vi "Begin.vi"() -> (0 "error in":errorcluster)   [LabVIEW 2013]
doc: "Called before other user functions, this VI is expected to open initial I/O refnums, load in file data, and do all program initialization. Notice that the <B>error out</B> terminal is simply used for data flow. Wiring it to other structures or subVIs ensures that this VI runs first."
uses:
  <vilib>/Rock Robotics/WPI/Joystick/WPI_JoystickDeviceEnum.ctl
  <vilib>/Rock Robotics/SystemInterfaces/DIO/FPGA_DIOPWMChannel.ctl
  <vilib>/Rock Robotics/SystemInterfaces/AI/FPGA_AIChannel.ctl
  <vilib>/Rock Robotics/SystemInterfaces/Typedef/FPGA_TypedefAnalogModule.ctl
  <vilib>/Rock Robotics/SystemInterfaces/DIO/FPGA_DIOChannel.ctl
  <vilib>/Rock Robotics/WPI/Encoder/WPI_EncoderType.ctl
  <vilib>/Rock Robotics/WPI/RobotDrive/WPI_RobotDriveOpen2MotorWithTalon.vi
  <vilib>/Rock Robotics/WPI/MotorControl/WPI_MotorControlOpen Talon.vi
  <vilib>/Rock Robotics/WPI/Counter/WPI_CounterDigitalInputToDigitalSource.vi
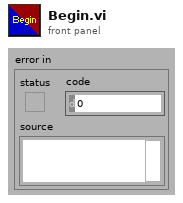
[diagram p1: front panel]
types:
  T1 = typedef "FPGA_DIOPWMChannel.ctl" = enum8{"PWM 1", "PWM 2", "PWM 3", "PWM 4", "PWM 5", "PWM 6", "PWM 7", "PWM 8", "PWM 9", "PWM 10", "Invalid"}
  T2 = typedef "WPI_JoystickDeviceEnum.ctl" = enum16{"USB 1", "USB 2", "USB 3", "USB 4", "Kinect 1", "Kinect 2"}
  T3 = typedef "FPGA_DIOChannel.ctl" = enum8{"DIO 1", "DIO 2", "DIO 3", "DIO 4", "DIO 5", "DIO 6", "DIO 7", "DIO 8", "DIO 9", "DIO 10", "DIO 11", "DIO 12", "DIO 13", "DIO 14", "Invalid"}
  T4 = typedef "WPI_EncoderType.ctl" = enum16{"1x", "2x", "4x"}
  T5 = typedef "FPGA_AIChannel.ctl" = enum8{"AI 1", "AI 2", "AI 3", "AI 4", "AI 5", "AI 6", "AI 7", "AI 8", "Invalid"}
  T6 = typedef "FPGA_TypedefAnalogModule.ctl" = enum16{"Analog Module 1", "Analog Module 2"}
  T7 = typedef "WPI_RobotDriveDevRef.ctl" = cluster{"DevStatus":errorcluster, "Motors[]":T8[], "Square Inputs":bool, "Max Output":dbl, "Isochronous":bool}
  T8 = typedef "WPI_MotorControlDeviceRef.ctl" = cluster{"DeviceStatus":errorcluster, "Type":enum16{"PWM", "CAN"}, "PWM":cluster{"Digital Module":T9, "PWM Channel":T1, "DeadBand":T10}, "CAN":cluster{"Device Number":u8, "Control Mode":T11, "Semaphore":T12, "Max Vout":dbl}, "Invert":bool, "TransformRef":T13, "InvTransformRef":T13}
  T9 = typedef "FPGA_TypedefDigitalModule.ctl" = enum16{"Digital Module 1", "Digital Module 2"}
  T10 = typedef "WPI_PWMDeadband.ctl" = cluster{"Name":string, "maxPositivePwm":i32, "minPositivePwm":i32, "centerPwm":i32, "maxNegativePwm":i32, "minNegativePwm":i32, "angularRange":u16}
  T11 = typedef "WPI_CANJaguar_ControlMode.ctl" = enum8{"Percent VBus", "Current", "Speed", "Position", "Voltage"}
  T12 = typedef "Semaphore RefNum" = refnum<k1>
  T13 = typedef "WPI_PWMTransform_ConPane.ctl" = refnum<vi>
  T14 = typedef "WPI_AnalogChannelDevRef.ctl" = cluster{"DevStatus":errorcluster, "Analog Module":T6, "Analog Channel":T5}
  T15 = typedef "WPI_DigitalInputDevRef.ctl" = cluster{"DevStatus":errorcluster, "DIO Channel":T3, "Digital Module":T9}
  T16 = typedef "FPGA_CounterEncoderSourceConvertionLVSourceType.ctl" = cluster{"DevStatus":errorcluster, "AnalogTriggerMode?":bool, "DigitalMode":cluster{"Digital Module":T9, "DIO Channel":T17}, "AnalogTriggerMode":cluster{"AnalogTriggerIndex":T18, "OutputType":T19}}
  T17 = typedef "FPGA_DIODigitalSourceChannel.ctl" = enum8{"DIO 1", "DIO 2", "DIO 3", "DIO 4", "DIO 5", "DIO 6", "DIO 7", "DIO 8", "DIO 9", "DIO 10", "DIO 11", "DIO 12", "DIO 13", "DIO 14", "Disabled"}
  T18 = typedef "FPGA_AnalogTriggerIndex.ctl" = enum8{"Trig 0", "Trig 1", "Trig 2", "Trig 3", "Trig 4", "Trig 5", "Trig 6", "Trig 7", "Invalid"}
  T19 = typedef "FPGA_AnalogTriggerOutType.ctl" = enum16{"InWindow", "TriggerState", "Rising", "Falling"}
  T20 = typedef "WPI_EncoderDevRef.ctl" = cluster{"DevStatus":errorcluster, "EncoderIndex":T21, "CounterIndex":T22, "DistancePerCount":dbl, "Decoding Type":T4}
  T21 = typedef "FPGA_EncoderIdx.ctl" = enum8{"Enc 0", "Enc 1", "Enc 2", "Enc 3", "Invalid"}
  T22 = typedef "FPGA_CounterCtrSystemIndex.ctl" = enum8{"Ctr 0", "Ctr 1", "Ctr 2", "Ctr 3", "Ctr 4", "Ctr 5", "Ctr 6", "Ctr 7", "Invalid"}
  T23 = typedef "WPI_JoystickDevRef.ctl" = cluster{"Device":T2}
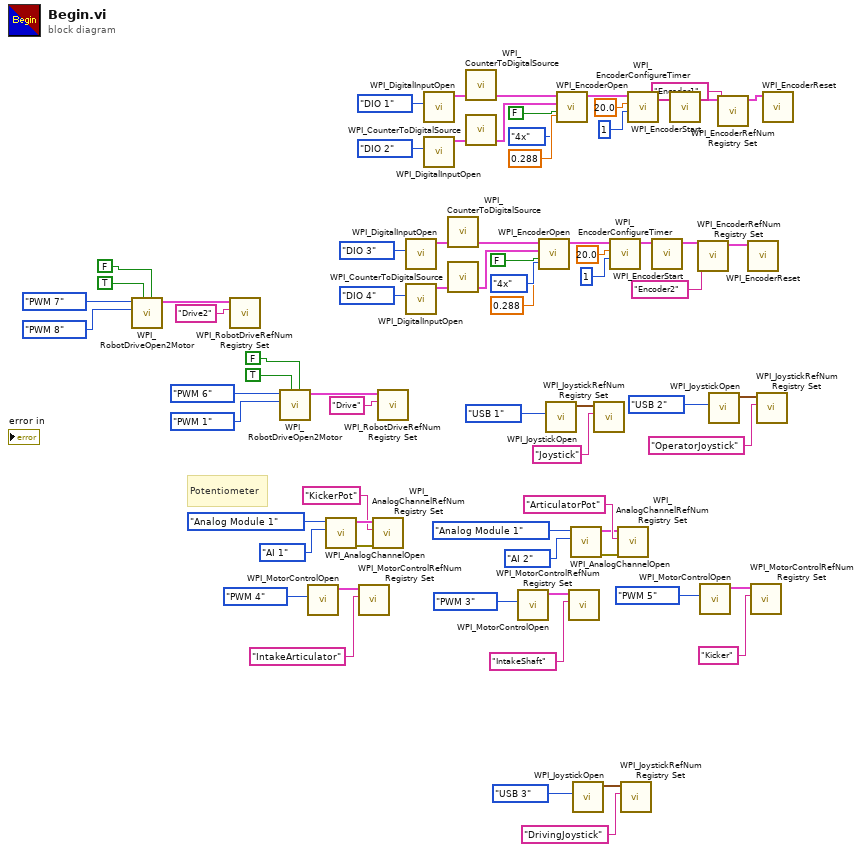
[diagram p0: block diagram]
diagram:
  # "Potentiometer"
  n1 = call-poly <vilib>:"WPI_RobotDriveOpen2Motor.vi"("Right Motor Inverted"=FALSE, "Left Motor Inverted"=TRUE, "Right Motor"=FPGA_DIOPWMChannel."PWM 8", "Left Motor"=FPGA_DIOPWMChannel."PWM 7") -> ("RobotDriveDevRef"=w68:T7)  [unwired: 6 in, 1 out]
  n2 = call <vilib>:"WPI_RobotDriveRefNum Registry Set.vi"("refnum name"="Drive2", "RobotDriveDevRef"=w68) -> ()  [unwired: 8 in, 2 out]
  n3 = call-poly <vilib>:"WPI_RobotDriveOpen2Motor.vi"("Right Motor Inverted"=FALSE, "Left Motor Inverted"=TRUE, "Right Motor"=FPGA_DIOPWMChannel."PWM 1", "Left Motor"=FPGA_DIOPWMChannel."PWM 6") -> ("RobotDriveDevRef"=w2:T7)  [unwired: 6 in, 1 out]
  n4 = call-poly <vilib>:"WPI_MotorControlOpen.vi"("PWM Channel"=FPGA_DIOPWMChannel."PWM 4") -> ("MotorControlDeviceRef"=w49:T8)  [unwired: 9 in, 1 out]
  n5 = call <vilib>:"WPI_AnalogChannelOpen.vi"("Analog Channel"=FPGA_AIChannel."AI 1", "Analog Module (Module 1)"=FPGA_TypedefAnalogModule."Analog Module 1") -> ("error out"=w58:errorcluster, "AIDeviceRef"=w57:T14)  [unwired: 8 in]
  n6 = call <vilib>:"WPI_MotorControlRefNum Registry Set.vi"("refnum name"="IntakeArticulator", "MotorControlDevRef"=w49) -> ()  [unwired: 8 in, 2 out]
  n7 = call <vilib>:"WPI_AnalogChannelRefNum Registry Set.vi"("error in (no error)"=w58, "refnum name"="KickerPot", "AIDeviceRef"=w57) -> ()  [unwired: 7 in, 2 out]
  n8 = call <vilib>:"WPI_RobotDriveRefNum Registry Set.vi"("refnum name"="Drive", "RobotDriveDevRef"=w2) -> ()  [unwired: 8 in, 2 out]
  n9 = call <vilib>:"WPI_DigitalInputOpen.vi"("DIO Channel"=FPGA_DIOChannel."DIO 3" ("Encoder A Channel")) -> ("DigitalInputDevRef"=w24:T15)  [unwired: 2 in, 8 out]
  n10 = call <vilib>:"WPI_DigitalInputOpen.vi"("DIO Channel"=FPGA_DIOChannel."DIO 4" ("Encoder B Channel")) -> ("DigitalInputDevRef"=w23:T15)  [unwired: 2 in, 8 out]
  n11 = call <vilib>:"WPI_DigitalInputOpen.vi"("DIO Channel"=FPGA_DIOChannel."DIO 1" ("Encoder A Channel")) -> ("DigitalInputDevRef"=w45:T15)  [unwired: 2 in, 8 out]
  n12 = call <vilib>:"WPI_DigitalInputOpen.vi"("DIO Channel"=FPGA_DIOChannel."DIO 2" ("Encoder B Channel")) -> ("DigitalInputDevRef"=w46:T15)  [unwired: 2 in, 8 out]
  n13 = call-poly <vilib>:"WPI_CounterToDigitalSource.vi"("DigitalInputDevRef"=w24) -> ("Digital Source"=w25:T16)  [unwired: 6 out]
  n14 = call-poly <vilib>:"WPI_CounterToDigitalSource.vi"("DigitalInputDevRef"=w23) -> ("Digital Source"=w22:T16)  [unwired: 6 out]
  n15 = call-poly <vilib>:"WPI_CounterToDigitalSource.vi"("DigitalInputDevRef"=w45) -> ("Digital Source"=w44:T16)  [unwired: 6 out]
  n16 = call-poly <vilib>:"WPI_CounterToDigitalSource.vi"("DigitalInputDevRef"=w46) -> ("Digital Source"=w47:T16)  [unwired: 6 out]
  n17 = call-poly <vilib>:"WPI_MotorControlOpen.vi"("PWM Channel"=FPGA_DIOPWMChannel."PWM 3") -> ("MotorControlDeviceRef"=w12:T8)  [unwired: 9 in, 1 out]
  n18 = call <vilib>:"WPI_EncoderOpen.vi"("DistancePerCount"=0.288 ("DistancePerCount (deg)"), "Decoding Type"=WPI_EncoderType."4x", "Invert Direction (False)"=FALSE ("Invert Direction"), "BSource"=w22, "ASource"=w25) -> ("EncoderDevRef"=w32:T20)  [unwired: 3 in, 3 out]
  n19 = call <vilib>:"WPI_JoystickOpen.vi"("JoystickDevice"=WPI_JoystickDeviceEnum."USB 1") -> ("JoystickDevRef"=w70:T23)  [unwired: 10 in]
  n20 = call <vilib>:"WPI_EncoderOpen.vi"("DistancePerCount"=0.288 ("DistancePerCount (deg)"), "Decoding Type"=WPI_EncoderType."4x", "Invert Direction (False)"=FALSE ("Invert Direction"), "BSource"=w47, "ASource"=w44) -> ("EncoderDevRef"=w37:T20)  [unwired: 3 in, 3 out]
  n21 = call <vilib>:"WPI_MotorControlRefNum Registry Set.vi"("refnum name"="IntakeShaft", "MotorControlDevRef"=w12) -> ()  [unwired: 8 in, 2 out]
  n22 = call <vilib>:"WPI_AnalogChannelOpen.vi"("Analog Channel"=FPGA_AIChannel."AI 2", "Analog Module (Module 1)"=FPGA_TypedefAnalogModule."Analog Module 1") -> ("error out"=w52:errorcluster, "AIDeviceRef"=w51:T14)  [unwired: 8 in]
  n23 = call <vilib>:"WPI_JoystickOpen.vi"("JoystickDevice"=WPI_JoystickDeviceEnum."USB 3") -> ("JoystickDevRef"=w8:T23)  [unwired: 10 in]
  n24 = call <vilib>:"WPI_JoystickRefNum Registry Set.vi"("refnum name"="Joystick", "JoystickDevRef"=w70) -> ()  [unwired: 8 in, 2 out]
  n25 = call <vilib>:"WPI_EncoderConfigureTimer.vi"("Number Samples to Average"=u8 1, "Minimum Rate"=20.0, "EncoderDevRef"=w32) -> ("EncoderDevRef"=w31:T20)  [unwired: 1 in, 7 out]
  n26 = call <vilib>:"WPI_AnalogChannelRefNum Registry Set.vi"("error in (no error)"=w52, "refnum name"="ArticulatorPot", "AIDeviceRef"=w51) -> ()  [unwired: 7 in, 2 out]
  n27 = call <vilib>:"WPI_JoystickRefNum Registry Set.vi"("refnum name"="DrivingJoystick", "JoystickDevRef"=w8) -> ()  [unwired: 8 in, 2 out]
  n28 = call <vilib>:"WPI_EncoderConfigureTimer.vi"("Number Samples to Average"=u8 1, "Minimum Rate"=20.0, "EncoderDevRef"=w37) -> ("EncoderDevRef"=w38:T20)  [unwired: 1 in, 7 out]
  n29 = call <vilib>:"WPI_EncoderStart.vi"("EncoderDevRef"=w31) -> ("EncoderDevRef"=w19:T20)  [unwired: 1 in, 9 out]
  n30 = call <vilib>:"WPI_EncoderStart.vi"("EncoderDevRef"=w38) -> ("EncoderDevRef"=w21:T20)  [unwired: 1 in, 9 out]
  n31 = call <vilib>:"WPI_EncoderRefNum Registry Set.vi"("refnum name"="Encoder2", "EncoderDevRef"=w19) -> ("EncoderDevRef"=w16:T20)  [unwired: 8 in, 1 out]
  n32 = call-poly <vilib>:"WPI_MotorControlOpen.vi"("PWM Channel"=FPGA_DIOPWMChannel."PWM 5") -> ("MotorControlDeviceRef"=w61:T8)  [unwired: 9 in, 1 out]
  n33 = call <vilib>:"WPI_JoystickOpen.vi"("JoystickDevice"=WPI_JoystickDeviceEnum."USB 2") -> ("JoystickDevRef"=w14:T23)  [unwired: 10 in]
  n34 = call <vilib>:"WPI_EncoderRefNum Registry Set.vi"("refnum name"="Encoder1", "EncoderDevRef"=w21) -> ("EncoderDevRef"=w17:T20)  [unwired: 8 in, 1 out]
  n35 = call <vilib>:"WPI_EncoderReset.vi"("EncoderDevRef"=w16) -> ()  [unwired: 9 in, 2 out]
  n36 = call <vilib>:"WPI_MotorControlRefNum Registry Set.vi"("refnum name"="Kicker", "MotorControlDevRef"=w61) -> ()  [unwired: 8 in, 2 out]
  n37 = call <vilib>:"WPI_JoystickRefNum Registry Set.vi"("refnum name"="OperatorJoystick", "JoystickDevRef"=w14) -> ()  [unwired: 8 in, 2 out]
  n38 = call <vilib>:"WPI_EncoderReset.vi"("EncoderDevRef"=w17) -> ()  [unwired: 9 in, 2 out]
